vi "Set Exposure.vi"(8 "error in (no error)":errorcluster, 10 "Exposure (ms)":u16) -> (0 "error out":errorcluster)   [LabVIEW 2015]
uses:
  HighFinesse WS5/HighFinesse WS5.lvlib
  HighFinesse WS5/wlmData.dll
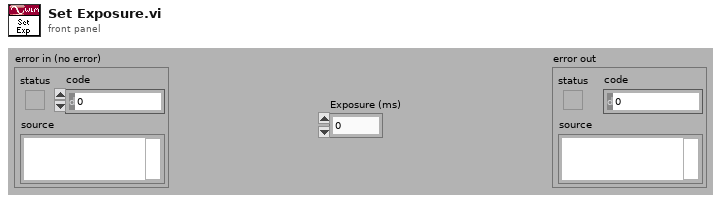
[diagram p1: front panel]
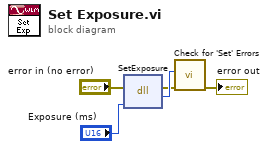
[diagram p0: block diagram]
diagram:
  n1 = dll-call lib="C:/LabVIEW-programs-dev/Instruments/Wavelength meter/HighFinesse WS5/wlmData.dll" fn="SetExposure"(error in="error in (no error)", "E"="Exposure (ms)") -> (error out=w2:errorcluster, "return type"=w3:i32)  [unwired: 3 in, 1 out]
  n2 = call "Check for 'Set' Errors.vi"("error in (no error)"=w2, "return value"=w3) -> ("error out"=→"error out":errorcluster)  [unwired: 8 in, 1 out]
